vi "Array of Variants to Array Variant.vi"(8 "error in (no error)":errorcluster, 11 "[Variant]":variant[](array[variant])) -> (0 "error out":errorcluster, 3 "Array Variant":variant)   [LabVIEW 2018, in "TwinCAT ADS.lvclass"]
uses:
  TwinCAT ADS.lvclass
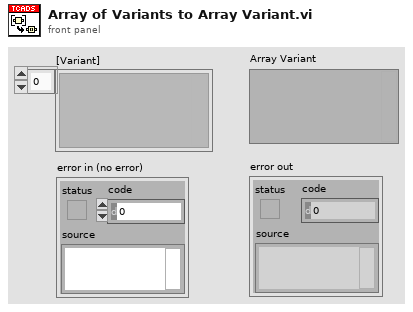
[diagram p1: front panel]
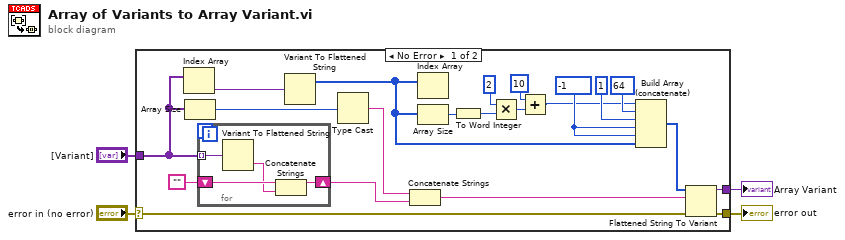
[diagram p0: block diagram]
diagram:
  n1 = case shown="No Error" "error in (no error)" {
    selector: "error in (no error)" -> [w20 w30]
    tunnel: [w19 w30] -> w3
    tunnel: "[Variant]" -> [w8 _]
    tunnel: [w18 _] -> w2
    frame No Error {
      w21 = i16 -1
      n2 = Index Array(array=w8) -> (element=w9:variant)  [unwired: 1 in]
      n3 = Array Size(array=w8) -> (size(s)=w7:i32)
      n4 = for {
        tunnel: w8 -> [w29] mode=indexing
        shift-right: [w27] -> w5
        shift-left: "" -> [w28]
        n5 = Variant To Flattened String(Variant=w29) -> (data string=w26:string)  [unwired: 1 out]
        n6 = Concatenate Strings(w28, w26) -> (w27:string)
      }
      n7 = Variant To Flattened String(Variant=w9) -> (1:w14:i16[])  [unwired: 1 out]
      n8 = Type Cast(x=w7) -> (*(type *) &x=w25:string)  [unwired: 1 in]
      n9 = Concatenate Strings(w25, w5) -> (w17:string)
      n10 = Index Array(array=w14) -> ()  [unwired: 1 in, 1 out]
      n11 = Array Size(array=w14) -> (size(s)=w24:i32)
      n12 = To Word Integer(number=w24) -> (16bit integer=w11:i16)
      n13 = Multiply(x=i16 2, y=w11) -> (x*y=w13:i16)
      n14 = Add(x=i16 10, y=w13) -> (x+y=w15:i16)
      n15 = Build Array (concatenate)(w15, i16 64, i16 1 ("element"), w21, w21, w14) -> (w12:i16[])
      n16 = Flattened String To Variant(4:w20, 6:w17, 7:w12) -> (0:w19:errorcluster, 3:w18:variant)
    }
    frame Error {
    }
  }
  "error out" <- w3
  "Array Variant" <- w2
